vi "FTDI_Kharonvi.vi"(8 "error in (no error)":errorcluster={"status"=FALSE, "code"=5000, "source"="Warning: Subvi \"Instrument_Error_Msg.vi\" not defined for instrument \"K2450\"\nSource: warn_about_missing_instrument.vi->Instrument_Error_Msg.vi->Reset all instruments.vi->Init Method V2.vi->Init_Everything.vi->ADC Int Ref Variation.vi\r\n"}, 11 "EM Slot":string="3") -> (0 "Error Out":errorcluster={"status"=FALSE, "code"=5000, "source"="Warning: Subvi \"Instrument_Error_Msg.vi\" not defined for instrument \"K2450\"\nSource: warn_about_missing_instrument.vi->Instrument_Error_Msg.vi->Reset all instruments.vi->Init Method V2.vi->Init_Everything.vi->ADC Int Ref Variation.vi\r\n"})   [LabVIEW 2019]
uses:
  <userlib>/_TI-LA/Instr Drivers/USB Interface/FTDI/Driver/FTDI.lvlib
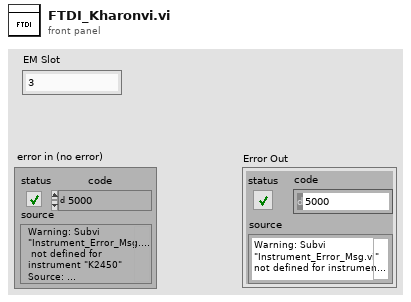
[diagram p1: front panel]
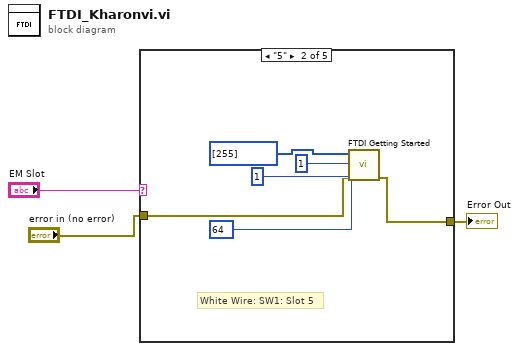
[diagram p0: block diagram]
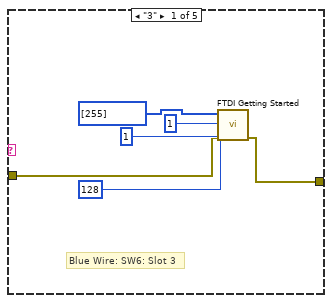
[diagram p2: hidden frame]
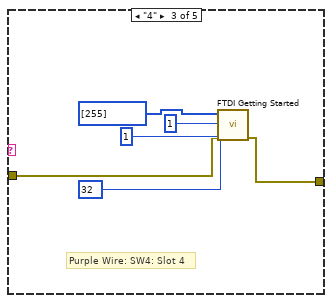
[diagram p3: hidden frame]
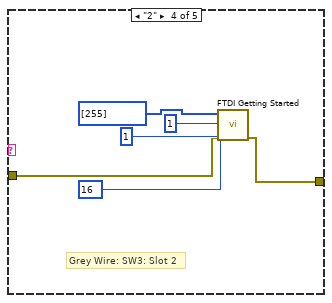
[diagram p4: hidden frame]
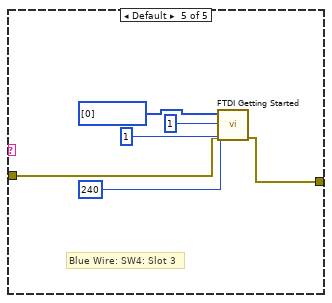
[diagram p5: hidden frame]
diagram:
  n1 = case shown="\"5\"" "EM Slot" {
    tunnel: "error in (no error)" -> [w5 w11 w17 w23 w29]
    tunnel: [w4 w10 w16 w22 w28] -> w2
    frame "3" {
      # "Blue Wire: SW6: Slot 3"
      n2 = call <userlib>:"FTDI Getting Started.vi"("Data[]"=u8[] [255], "Device Index"=u32 1, "Bit Mode"=u8 1, "IO Mask (1 = Output)"=u8 128, "Error In"=w5) -> ("Error Out"=w4:errorcluster)  [unwired: 9 in, 1 out]
    }
    frame "5" {
      # "White Wire: SW1: Slot 5"
      n3 = call <userlib>:"FTDI Getting Started.vi"("Data[]"=u8[] [255], "Device Index"=u32 1, "Bit Mode"=u8 1, "IO Mask (1 = Output)"=u8 64, "Error In"=w11) -> ("Error Out"=w10:errorcluster)  [unwired: 9 in, 1 out]
    }
    frame "4" {
      # "Purple Wire: SW4: Slot 4"
      n4 = call <userlib>:"FTDI Getting Started.vi"("Data[]"=u8[] [255], "Device Index"=u32 1, "Bit Mode"=u8 1, "IO Mask (1 = Output)"=u8 32, "Error In"=w17) -> ("Error Out"=w16:errorcluster)  [unwired: 9 in, 1 out]
    }
    frame "2" {
      # "Grey Wire: SW3: Slot 2"
      n5 = call <userlib>:"FTDI Getting Started.vi"("Data[]"=u8[] [255], "Device Index"=u32 1, "Bit Mode"=u8 1, "IO Mask (1 = Output)"=u8 16, "Error In"=w23) -> ("Error Out"=w22:errorcluster)  [unwired: 9 in, 1 out]
    }
    frame Default {
      # "Blue Wire: SW4: Slot 3"
      n6 = call <userlib>:"FTDI Getting Started.vi"("Data[]"=u8[] [0], "Device Index"=u32 1, "Bit Mode"=u8 1, "IO Mask (1 = Output)"=u8 240, "Error In"=w29) -> ("Error Out"=w28:errorcluster)  [unwired: 9 in, 1 out]
    }
  }
  "Error Out" <- w2
